vi "Initialize DI.vi"(8 "error in (no error)":errorcluster, 9 "DI Channel Setting":T1, 10 "DAQ Type":enum16{"Hardware", "Simulation"}(ring), 11 "Abstract in":refnum<class "Abstract.lvclass">) -> (0 "error out":errorcluster, 3 "Abstract out":refnum<class "Abstract.lvclass">)   [LabVIEW 2021, in "DAQ IO.lvlib" / "Abstract.lvclass"]
uses:
  Abstract.lvclass
  DI Channel Setting.ctl
  DAQ IO.lvlib
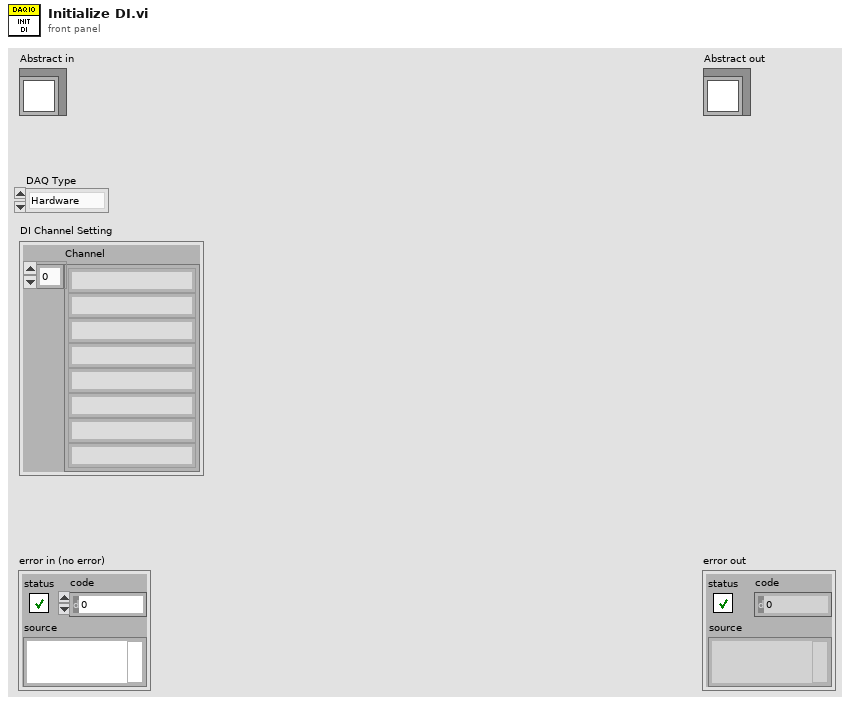
[diagram p1: front panel]
types:
  T1 = typedef "DAQ IO.lvlib/DI Channel Setting.ctl" = cluster{"Channel":string[]}
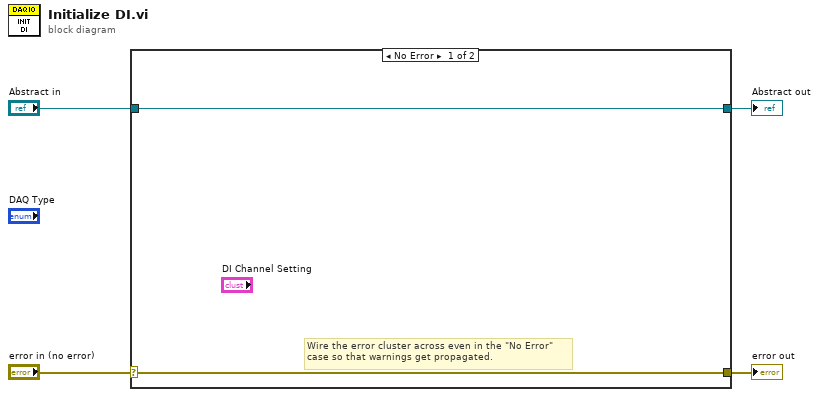
[diagram p0: block diagram]
diagram:
  n1 = case shown="No Error" "error in (no error)" {
    selector: "error in (no error)" -> [w5 w8]
    tunnel: [w5 w8] -> w3
    tunnel: [w6 w7] -> w1
    tunnel: "Abstract in" -> [w6 w7]
    frame No Error {
      # "Wire the error cluster across even in the \"No Error\"\ncase so that warnings get propagated."
    }
    frame Error {
    }
  }
  "error out" <- w3
  "Abstract out" <- w1
